vi "AuMT8852B Modulation Index Test Configuration.vi"(5 "Settings":T1={"Low frequency selection"=enum."Use low frequency", "Medium frequency selection"=enum."Use medium frequency", "High frequency selection"=enum."Use high frequency", "Low TX frequency"=2402.0, "Low RX frequency"=2480.0, "Medium TX frequency"=2441.0, "Medium RX frequency"=2402.0, "High TX frequency"=2480.0, "High RX frequency"=2402.0, "Number of packets"=10, "f1 average minimum"=140000.0, "f1 average maximum"=175000.0, "f2 maximum limit"=115000.0, "f1/f2 average maximum"=0.8, "Test control"=enum."Loopback", "Packet type"=enum."Longest supported", "Change payload"=enum."Once"} {"f1/f2 average maximum" format="%.1f"}, 7 "Set/Get (Set)":enum16{"Set", "Get"}(ring), 8 "error in (no error)":errorcluster, 10 "Script (3)":i32=3, 11 "VISA session":refnum<visa-resource-name>) -> (0 "error out":errorcluster, 2 "error code":i32, 3 "VISA session out":refnum<visa-resource-name>, 4 "Settings out":T1={"Low frequency selection"=enum."Use low frequency", "Medium frequency selection"=enum."Use medium frequency", "High frequency selection"=enum."Use high frequency", "Low TX frequency"=2402.0, "Low RX frequency"=2480.0, "Medium TX frequency"=2441.0, "Medium RX frequency"=2402.0, "High TX frequency"=2480.0, "High RX frequency"=2402.0, "Number of packets"=10, "f1 average minimum"=140000.0, "f1 average maximum"=175000.0, "f2 maximum limit"=115000.0, "f1/f2 average maximum"=0.8, "Test control"=enum."Loopback", "Packet type"=enum."Longest supported", "Change payload"=enum."Once"} {"f1/f2 average maximum" format="%.1f"})   [LabVIEW 2017]
doc: "Anritsu MT8852B Bluetooth Tester\n\nConfigures the instrument for the Modulation Characteristics test.\n\nINPUTS\nSet/Get - whether the values are being sent to or retrieved from the instrument.\nScript - which of the stored scripts (1-10) will be queried or configured. Scripts 1 and 2 are read-only.\nSettings - parameters of the test to be written.\n\nOUTPUTS\nSettings out - current parameters of the test."
uses:
  <instrlib>/aumt8852B/General/Utilities/MT8850 Test Parameters.ctl
  <instrlib>/aumt8852B/General/Utilities/MT8850 Frequency Units.ctl
panel:
  in  "Case Constant\n(See Context Help)":bool
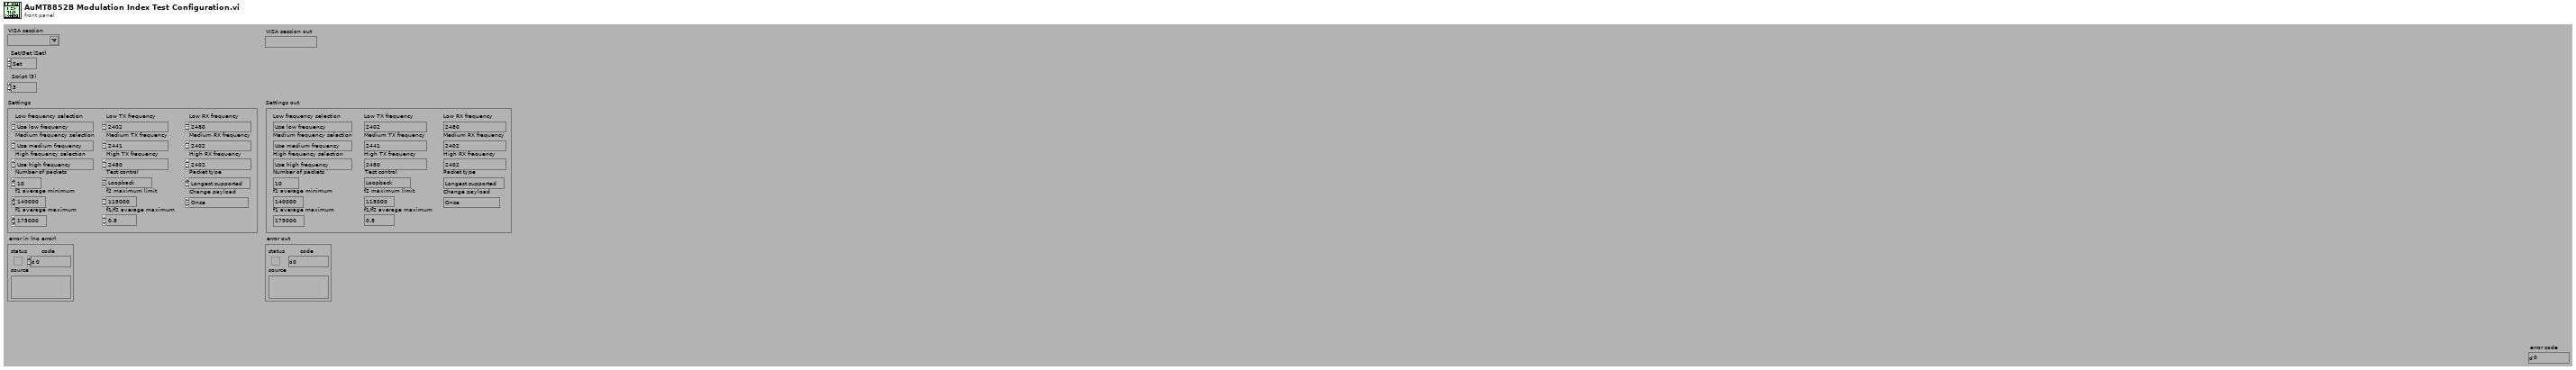
[diagram p1: front panel]
types:
  T1 = cluster{"Low frequency selection":enum16{"Don't use low frequency", "Use low frequency"}, "Medium frequency selection":enum16{"Don't use medium frequency", "Use medium frequency"}, "High frequency selection":enum16{"Don't use high frequency", "Use high frequency"}, "Low TX frequency":dbl, "Low RX frequency":dbl, "Medium TX frequency":dbl, "Medium RX frequency":dbl, "High TX frequency":dbl, "High RX frequency":dbl, "Number of packets":i32, "f1 average minimum":dbl, "f1 average maximum":dbl, "f2 maximum limit":dbl, "f1/f2 average maximum":dbl, "Test control":enum16{"Loopback", "TX test"}, "Packet type":enum16{"Longest supported", "DH5", "DH3", "DH1"}, "Change payload":enum16{"Once", "Continuous"}}
  T2 = typedef "MT8850 Test Parameters.ctl" = enum16{"Use low frequency", "Use medium frequency", "Use high frequency", "Low TX frequency", "Low RX frquency", "Medium TX frequency", "Medium RX frequency", "High TX frequency", "High RX frequency", "Number of packets", "Average high limit", "Average low limit", "Peak power limit", "Max power step limit", "Min power step limit", "f1 average minimum", "f1 average maximum", "f2 maximum", "f1/f2 average maximum", "Hop selection", "Use DH1 packets", "Use DH3 packets", "Use DH5 packets", "1 slot packet drift limit", "3 slot packet drift limit", "5 slot packet drift limit", "Drift rate limit", "TX power level", "Frequency offset", "Symbol timing", "Modulation index", "BER limit", "FER limit", "Use averaging high limit", "Use averaging low limit", "Use peak power limit", "Packet type", "Test control", "Use max power step limit", "Use min power step limit", "Number of cycles", "Use f1 average maximum", "Use f1 average minimum", "Use f2 maximum", "Use f1/f2 average maximum", "Hop mode", "Maximum negative limit", "Maximum positive limit", "Use maximum negative limit", "Use maximum positive limit", "Use 1 slot packet drift limit", "Use 3 slot packet drift limit", "Use 5 slot packet drift limit", "Use drift rate limit", "Use BER limit", "Use FER limit", "Use dirty parameter table", "Use null packet drift limit", "Null packet drift limit", "Minimum power", "Power delay", "Packet count", "Payload toggle", "Output power level", "2DHX packet type", "3DHX packet type", "Number of blocks", "TX and RX low frequency", "TX and RX medium frequency", "TX and RX high frequency", "TX frequency", "RX frequency", "Threshold bit count", "Total test bit count", "Number of bits", "PDPSK to PGFSK lower limit", "PDPSK to PGFSK upper limit", "Initial frequency error upper limit", "Initial frequency error lower limit", "Frequency error upper limit", "Frequency error lower limit", "Block frequency error upper limit", "Block frequency error lower limit", "2Mbs RMS DEVM limit", "3Mbs RMS DEVM limit", "2Mbs Peak DEVM limit", "3Mbs Peak DEVM limit", "2Mbs 99% packets DEVM limit", "3Mbs 99% packets DEVM limit", "Percentage of no error packets limit", "Threshold error limit", "Total test error limit"}
  T3 = typedef "MT8850 Frequency Units.ctl" = enum16{"Channel", "Hz", "kHz", "MHz", "GHz"}
  T4 = enum16{"Simulate", "Range check", "Cache", "Query instrument status"}
  T5 = enum16{"Output power", "Power control", "Modulation characteristics", "Initial carrier", "Carrier drift", "Single slot sensitivity", "Multiple slot sensitivity", "Maximum input power"}
  T6 = enum16{"Don't use high frequency", "Use high frequency"}
  T7 = enum16{"Don't use medium frequency", "Use medium frequency"}
  T8 = enum16{"Don't use low frequency", "Use low frequency"}
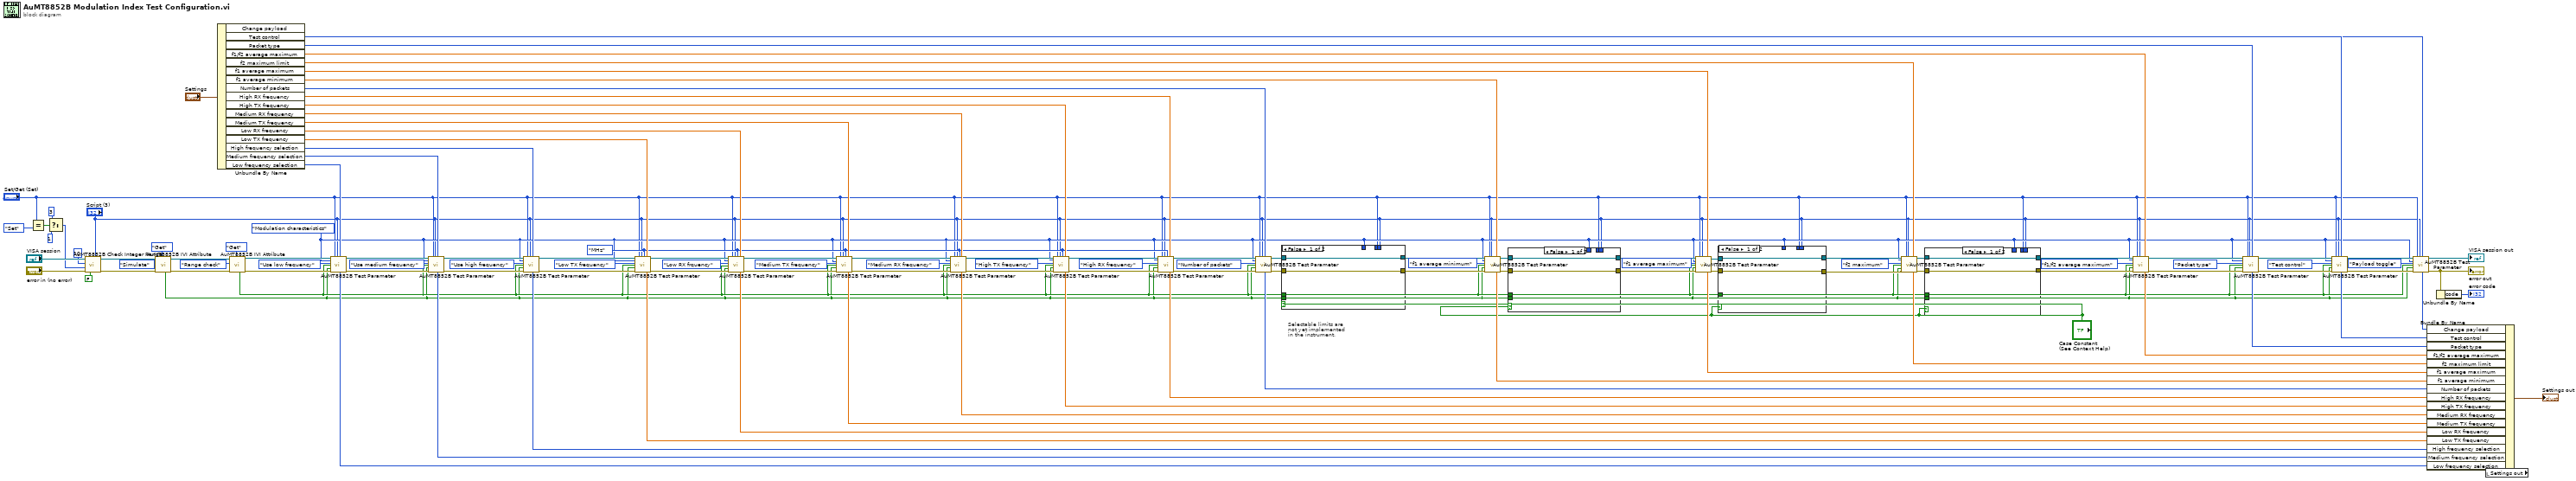
[diagram p0: block diagram]
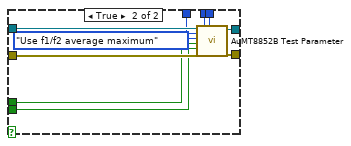
[diagram p2: hidden frame]
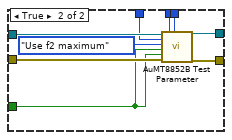
[diagram p3: hidden frame]
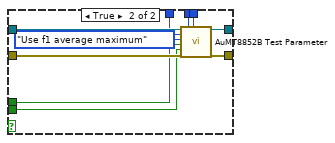
[diagram p4: hidden frame]
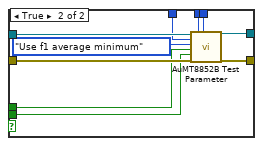
[diagram p5: hidden frame]
diagram:
  w13 = MT8850_Frequency_Units."MHz" ("Frequency units (MHz)")
  w8 = T5."Modulation characteristics" ("Test (Output Power)")
  # "Selectable limits are\nnot yet implemented\nin the instrument."
  n1 = Equal?(x="Set/Get (Set)", y=enum16{"Set", "Get"}."Set") -> (x = y?=w120:bool)
  n2 = Select(t=3, s=w120, f=1) -> (s? t:f=w116:i32)
  n3 = call <instrlib>:"AuMT8852B Check Integer Range.vi"("Value (0)"="Script (3)", "Check IVI flag first? (T)"=FALSE, "error in (no error)"="error in (no error)", "Lower limit (-1)"=w116, "Upper limit (1)"=10, "VISA session"="VISA session") -> ("error out"=w114:errorcluster, "VISA session out"=w115:refnum<visa-resource-name>)  [unwired: 4 in]
  n4 = call <instrlib>:"AuMT8852B IVI Attribute.vi"("Set/Get (Set)"=enum16{"Set", "Get"}."Get", "error in (no error)"=w114, "Flag (Simulate)"=T4."Simulate", "VISA session"=w115) -> ("error out"=w88:errorcluster, "VISA session out"=w89:refnum<visa-resource-name>, "Value out"=w5:bool)  [unwired: 5 in]
  n5 = Unbundle By Name("Settings") -> ("Change payload"=w1:enum16{"Once", "Continuous"}, "Test control"=w40:enum16{"Loopback", "TX test"}, "Packet type"=w41:enum16{"Longest supported", "DH5", "DH3", "DH1"}, "f1/f2 average maximum"=w56:dbl, "f2 maximum limit"=w55:dbl, "f1 average maximum"=w58:dbl, "f1 average minimum"=w59:dbl, "Number of packets"=w60:i32, "High RX frequency"=w75:dbl, "High TX frequency"=w76:dbl, "Medium RX frequency"=w61:dbl, "Medium TX frequency"=w77:dbl, "Low RX frequency"=w78:dbl, "Low TX frequency"=w79:dbl, "High frequency selection"=w80:T6, "Medium frequency selection"=w81:T7, "Low frequency selection"=w82:T8)
  n6 = call <instrlib>:"AuMT8852B IVI Attribute.vi"("Set/Get (Set)"=enum16{"Set", "Get"}."Get", "error in (no error)"=w88, "Flag (Simulate)"=T4."Range check", "VISA session"=w89) -> ("error out"=w86:errorcluster, "VISA session out"=w87:refnum<visa-resource-name>, "Value out"=w6:bool)  [unwired: 5 in]
  n7 = call <instrlib>:"AuMT8852B Test Parameter.vi"("VISA session"=w87, "Test (Output power)"=w8, "Parameter (Use low frequency)"=MT8850_Test_Parameters."Use low frequency", "Range check? (F)"=w6, "Simulate? (F)"=w5, "error in (no error)"=w86, "Set/Get (Set)"="Set/Get (Set)", "Script (3)"="Script (3)", "Integer value (0)"=w82) -> ("Integer value out"=w67:i32, "VISA session out"=w20:refnum<visa-resource-name>, "error out"=w19:errorcluster)  [unwired: 7 in, 1 out]
  n8 = call <instrlib>:"AuMT8852B Test Parameter.vi"("VISA session"=w20, "Test (Output power)"=w8, "Parameter (Use low frequency)"=MT8850_Test_Parameters."Use medium frequency", "Range check? (F)"=w6, "Simulate? (F)"=w5, "error in (no error)"=w19, "Set/Get (Set)"="Set/Get (Set)", "Script (3)"="Script (3)", "Integer value (0)"=w81) -> ("Integer value out"=w68:i32, "VISA session out"=w18:refnum<visa-resource-name>, "error out"=w17:errorcluster)  [unwired: 7 in, 1 out]
  n9 = call <instrlib>:"AuMT8852B Test Parameter.vi"("VISA session"=w18, "Test (Output power)"=w8, "Parameter (Use low frequency)"=MT8850_Test_Parameters."Use high frequency", "Range check? (F)"=w6, "Simulate? (F)"=w5, "error in (no error)"=w17, "Set/Get (Set)"="Set/Get (Set)", "Script (3)"="Script (3)", "Integer value (0)"=w80) -> ("Integer value out"=w69:i32, "VISA session out"=w110:refnum<visa-resource-name>, "error out"=w109:errorcluster)  [unwired: 7 in, 1 out]
  n10 = call <instrlib>:"AuMT8852B Test Parameter.vi"("VISA session"=w110, "Test (Output power)"=w8, "Parameter (Use low frequency)"=MT8850_Test_Parameters."Low TX frequency", "Range check? (F)"=w6, "Simulate? (F)"=w5, "error in (no error)"=w109, "Set/Get (Set)"="Set/Get (Set)", "Script (3)"="Script (3)", "Integer value (0)"=w13, "Float value (0)"=w79) -> ("Float value out"=w70:dbl, "VISA session out"=w108:refnum<visa-resource-name>, "error out"=w107:errorcluster)  [unwired: 6 in, 1 out]
  n11 = call <instrlib>:"AuMT8852B Test Parameter.vi"("VISA session"=w108, "Test (Output power)"=w8, "Parameter (Use low frequency)"=MT8850_Test_Parameters."Low RX frquency", "Range check? (F)"=w6, "Simulate? (F)"=w5, "error in (no error)"=w107, "Set/Get (Set)"="Set/Get (Set)", "Script (3)"="Script (3)", "Integer value (0)"=w13, "Float value (0)"=w78) -> ("Float value out"=w71:dbl, "VISA session out"=w106:refnum<visa-resource-name>, "error out"=w105:errorcluster)  [unwired: 6 in, 1 out]
  n12 = call <instrlib>:"AuMT8852B Test Parameter.vi"("VISA session"=w106, "Test (Output power)"=w8, "Parameter (Use low frequency)"=MT8850_Test_Parameters."Medium TX frequency", "Range check? (F)"=w6, "Simulate? (F)"=w5, "error in (no error)"=w105, "Set/Get (Set)"="Set/Get (Set)", "Script (3)"="Script (3)", "Integer value (0)"=w13, "Float value (0)"=w77) -> ("Float value out"=w72:dbl, "VISA session out"=w104:refnum<visa-resource-name>, "error out"=w103:errorcluster)  [unwired: 6 in, 1 out]
  n13 = call <instrlib>:"AuMT8852B Test Parameter.vi"("VISA session"=w104, "Test (Output power)"=w8, "Parameter (Use low frequency)"=MT8850_Test_Parameters."Medium RX frequency", "Range check? (F)"=w6, "Simulate? (F)"=w5, "error in (no error)"=w103, "Set/Get (Set)"="Set/Get (Set)", "Script (3)"="Script (3)", "Integer value (0)"=w13, "Float value (0)"=w61) -> ("Float value out"=w65:dbl, "VISA session out"=w102:refnum<visa-resource-name>, "error out"=w101:errorcluster)  [unwired: 6 in, 1 out]
  n14 = call <instrlib>:"AuMT8852B Test Parameter.vi"("VISA session"=w102, "Test (Output power)"=w8, "Parameter (Use low frequency)"=MT8850_Test_Parameters."High TX frequency", "Range check? (F)"=w6, "Simulate? (F)"=w5, "error in (no error)"=w101, "Set/Get (Set)"="Set/Get (Set)", "Script (3)"="Script (3)", "Integer value (0)"=w13, "Float value (0)"=w76) -> ("Float value out"=w73:dbl, "VISA session out"=w100:refnum<visa-resource-name>, "error out"=w99:errorcluster)  [unwired: 6 in, 1 out]
  n15 = call <instrlib>:"AuMT8852B Test Parameter.vi"("VISA session"=w100, "Test (Output power)"=w8, "Parameter (Use low frequency)"=MT8850_Test_Parameters."High RX frequency", "Range check? (F)"=w6, "Simulate? (F)"=w5, "error in (no error)"=w99, "Set/Get (Set)"="Set/Get (Set)", "Script (3)"="Script (3)", "Integer value (0)"=w13, "Float value (0)"=w75) -> ("Float value out"=w74:dbl, "VISA session out"=w98:refnum<visa-resource-name>, "error out"=w97:errorcluster)  [unwired: 6 in, 1 out]
  n16 = call <instrlib>:"AuMT8852B Test Parameter.vi"("VISA session"=w98, "Test (Output power)"=w8, "Parameter (Use low frequency)"=MT8850_Test_Parameters."Number of packets", "Range check? (F)"=w6, "Simulate? (F)"=w5, "error in (no error)"=w97, "Set/Get (Set)"="Set/Get (Set)", "Script (3)"="Script (3)", "Integer value (0)"=w60) -> ("Integer value out"=w64:i32, "VISA session out"=w24:refnum<visa-resource-name>, "error out"=w23:errorcluster)  [unwired: 7 in, 1 out]
  n17 = case shown="False" "Case Constant\n(See Context Help)" {
    tunnel: [w124 w134] -> w26
    tunnel: [w125 w133] -> w25
    tunnel: w24 -> [w125 w132]
    tunnel: w23 -> [w124 w131]
    tunnel: w6 -> [_ w130]
    tunnel: w5 -> [_ w129]
    tunnel: w8 -> [_ w128]
    tunnel: "Set/Get (Set)" -> [_ w127]
    tunnel: "Script (3)" -> [_ w126]
    frame False {
    }
    frame True {
      n18 = call <instrlib>:"AuMT8852B Test Parameter.vi"("VISA session"=w132, "Test (Output power)"=w128, "Parameter (Use low frequency)"=MT8850_Test_Parameters."Use f1 average minimum", "Range check? (F)"=w130, "Simulate? (F)"=w129, "error in (no error)"=w131, "Set/Get (Set)"=w127, "Script (3)"=w126) -> ("VISA session out"=w133:refnum<visa-resource-name>, "error out"=w134:errorcluster)  [unwired: 8 in, 2 out]
    }
  }
  n19 = call <instrlib>:"AuMT8852B Test Parameter.vi"("VISA session"=w25, "Test (Output power)"=w8, "Parameter (Use low frequency)"=MT8850_Test_Parameters."f1 average minimum", "Range check? (F)"=w6, "Simulate? (F)"=w5, "error in (no error)"=w26, "Set/Get (Set)"="Set/Get (Set)", "Script (3)"="Script (3)", "Float value (0)"=w59) -> ("Float value out"=w63:dbl, "VISA session out"=w28:refnum<visa-resource-name>, "error out"=w30:errorcluster)  [unwired: 7 in, 1 out]
  n20 = case shown="False" "Case Constant\n(See Context Help)" {
    tunnel: w30 -> [w137 w146]
    tunnel: [w137 w145] -> w29
    tunnel: w28 -> [w136 w144]
    tunnel: [w136 w143] -> w27
    tunnel: w6 -> [_ w142]
    tunnel: w5 -> [_ w141]
    tunnel: w8 -> [_ w140]
    tunnel: "Set/Get (Set)" -> [_ w139]
    tunnel: "Script (3)" -> [_ w138]
    frame False {
    }
    frame True {
      n21 = call <instrlib>:"AuMT8852B Test Parameter.vi"("VISA session"=w144, "Test (Output power)"=w140, "Parameter (Use low frequency)"=MT8850_Test_Parameters."Use f1 average maximum", "Range check? (F)"=w142, "Simulate? (F)"=w141, "error in (no error)"=w146, "Set/Get (Set)"=w139, "Script (3)"=w138) -> ("VISA session out"=w143:refnum<visa-resource-name>, "error out"=w145:errorcluster)  [unwired: 8 in, 2 out]
    }
  }
  n22 = call <instrlib>:"AuMT8852B Test Parameter.vi"("VISA session"=w27, "Test (Output power)"=w8, "Parameter (Use low frequency)"=MT8850_Test_Parameters."f1 average maximum", "Range check? (F)"=w6, "Simulate? (F)"=w5, "error in (no error)"=w29, "Set/Get (Set)"="Set/Get (Set)", "Script (3)"="Script (3)", "Float value (0)"=w58) -> ("Float value out"=w62:dbl, "VISA session out"=w32:refnum<visa-resource-name>, "error out"=w35:errorcluster)  [unwired: 7 in, 1 out]
  n23 = case shown="False" "Case Constant\n(See Context Help)" {
    tunnel: w35 -> [w148 w157]
    tunnel: [w148 w156] -> w34
    tunnel: [w149 w155] -> w33
    tunnel: w32 -> [w149 w154]
    tunnel: w6 -> [_ w153]
    tunnel: w8 -> [_ w152]
    tunnel: "Set/Get (Set)" -> [_ w151]
    tunnel: "Script (3)" -> [_ w150]
    frame False {
    }
    frame True {
      n24 = call <instrlib>:"AuMT8852B Test Parameter.vi"("VISA session"=w154, "Test (Output power)"=w152, "Parameter (Use low frequency)"=MT8850_Test_Parameters."Use f2 maximum", "Range check? (F)"=w153, "Simulate? (F)"=w153, "error in (no error)"=w157, "Set/Get (Set)"=w151, "Script (3)"=w150) -> ("VISA session out"=w155:refnum<visa-resource-name>, "error out"=w156:errorcluster)  [unwired: 8 in, 2 out]
    }
  }
  n25 = call <instrlib>:"AuMT8852B Test Parameter.vi"("VISA session"=w33, "Test (Output power)"=w8, "Parameter (Use low frequency)"=MT8850_Test_Parameters."f2 maximum", "Range check? (F)"=w6, "Simulate? (F)"=w5, "error in (no error)"=w34, "Set/Get (Set)"="Set/Get (Set)", "Script (3)"="Script (3)", "Float value (0)"=w55) -> ("Float value out"=w50:dbl, "VISA session out"=w36:refnum<visa-resource-name>, "error out"=w39:errorcluster)  [unwired: 7 in, 1 out]
  n26 = case shown="False" "Case Constant\n(See Context Help)" {
    tunnel: w39 -> [w159 w169]
    tunnel: [w159 w168] -> w38
    tunnel: [w160 w167] -> w37
    tunnel: w36 -> [w160 w166]
    tunnel: w6 -> [_ w165]
    tunnel: w5 -> [_ w164]
    tunnel: w8 -> [_ w163]
    tunnel: "Set/Get (Set)" -> [_ w162]
    tunnel: "Script (3)" -> [_ w161]
    frame False {
    }
    frame True {
      n27 = call <instrlib>:"AuMT8852B Test Parameter.vi"("VISA session"=w166, "Test (Output power)"=w163, "Parameter (Use low frequency)"=MT8850_Test_Parameters."Use f1/f2 average maximum", "Range check? (F)"=w165, "Simulate? (F)"=w164, "error in (no error)"=w169, "Set/Get (Set)"=w162, "Script (3)"=w161) -> ("VISA session out"=w167:refnum<visa-resource-name>, "error out"=w168:errorcluster)  [unwired: 8 in, 2 out]
    }
  }
  n28 = call <instrlib>:"AuMT8852B Test Parameter.vi"("VISA session"=w37, "Test (Output power)"=w8, "Parameter (Use low frequency)"=MT8850_Test_Parameters."f1/f2 average maximum", "Range check? (F)"=w6, "Simulate? (F)"=w5, "error in (no error)"=w38, "Set/Get (Set)"="Set/Get (Set)", "Script (3)"="Script (3)", "Float value (0)"=w56) -> ("Float value out"=w51:dbl, "VISA session out"=w46:refnum<visa-resource-name>, "error out"=w47:errorcluster)  [unwired: 7 in, 1 out]
  n29 = call <instrlib>:"AuMT8852B Test Parameter.vi"("VISA session"=w46, "Test (Output power)"=w8, "Parameter (Use low frequency)"=MT8850_Test_Parameters."Packet type", "Range check? (F)"=w6, "Simulate? (F)"=w5, "error in (no error)"=w47, "Set/Get (Set)"="Set/Get (Set)", "Script (3)"="Script (3)", "Integer value (0)"=w41) -> ("Integer value out"=w42:i32, "VISA session out"=w45:refnum<visa-resource-name>, "error out"=w44:errorcluster)  [unwired: 7 in, 1 out]
  n30 = call <instrlib>:"AuMT8852B Test Parameter.vi"("VISA session"=w45, "Test (Output power)"=w8, "Parameter (Use low frequency)"=MT8850_Test_Parameters."Test control", "Range check? (F)"=w6, "Simulate? (F)"=w5, "error in (no error)"=w44, "Set/Get (Set)"="Set/Get (Set)", "Script (3)"="Script (3)", "Integer value (0)"=w40) -> ("Integer value out"=w43:i32, "VISA session out"=w12:refnum<visa-resource-name>, "error out"=w11:errorcluster)  [unwired: 7 in, 1 out]
  n31 = call <instrlib>:"AuMT8852B Test Parameter.vi"("VISA session"=w12, "Test (Output power)"=w8, "Parameter (Use low frequency)"=MT8850_Test_Parameters."Payload toggle", "Range check? (F)"=w6, "Simulate? (F)"=w5, "error in (no error)"=w11, "Set/Get (Set)"="Set/Get (Set)", "Script (3)"="Script (3)", "Integer value (0)"=w1) -> ("Integer value out"=w4:i32, "VISA session out"=→"VISA session out":refnum<visa-resource-name>, "error out"=w10:errorcluster)  [unwired: 7 in, 1 out]
  "error out" <- w10
  n32 = Unbundle By Name(w10) -> ("code"=→"error code":i32)
  n33 = local read "Settings out"() -> (w66:T1)
  n34 = Bundle By Name(cluster=w66, "Change payload"=w4, "Test control"=w43, "Packet type"=w42, "f1/f2 average maximum"=w51, "f2 maximum limit"=w50, "f1 average maximum"=w62, "f1 average minimum"=w63, "Number of packets"=w64, "High RX frequency"=w74, "High TX frequency"=w73, "Medium RX frequency"=w65, "Medium TX frequency"=w72, "Low RX frequency"=w71, "Low TX frequency"=w70, "High frequency selection"=w69, "Medium frequency selection"=w68, "Low frequency selection"=w67) -> (→"Settings out":T1)
